vi "Test VI Inlining.vi"(8 "error in (no error)":errorcluster, 9 "Inline SubVI?":bool, 10 "VI Refnum":refnum<vi>, 11 "testStateMachineUtilities in":refnum<class "testStateMachineUtilities.lvclass">=refnum) -> (0 "error out":errorcluster, 3 "testStateMachineUtilities out":refnum<class "testStateMachineUtilities.lvclass">)   [LabVIEW 2016]
uses:
  testStateMachineUtilities/testStateMachineUtilities.lvclass
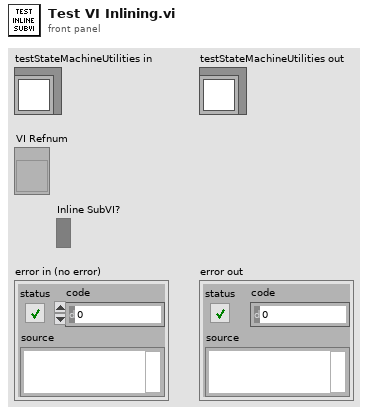
[diagram p1: front panel]
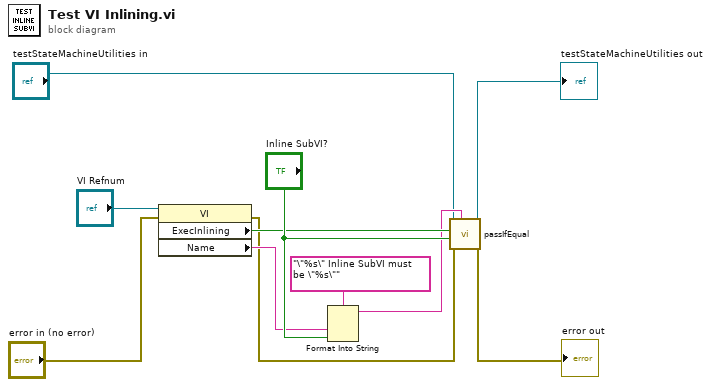
[diagram p0: block diagram]
diagram:
  n1 = property class="VI"(reference="VI Refnum", error in="error in (no error)") -> (error out=w8:errorcluster, "ExecInlining"=w10:bool, "Name"=w9:string)  [unwired: 1 out]
  n2 = Format Into String(format string="\"%s\" Inline SubVI must be \"%s\"", w9, "Inline SubVI?") -> (resulting string=w5:string)  [unwired: 2 in, 1 out]
  n3 = call-dynamic "passIfEqual.vi"("custom report message (\"\")"=w5, "error in (no error)"=w8, "y"="Inline SubVI?", "x"=w10, "TestCase in"="testStateMachineUtilities in") -> ("error out"=→"error out":errorcluster, "TestCase out"=→"testStateMachineUtilities out":refnum<class "testStateMachineUtilities.lvclass">)  [unwired: 5 in]
